vi "checkCmdIdRule.vi"(8 "error in (no error)":errorcluster, 10 "packetConnID":T1, 11 "tcpServer in":refnum<class "TcpServer.lvclass">) -> (0 "error out":errorcluster, 1 "ackIterations":i32, 2 "packetConnID":T1, 3 "tcpServer out":refnum<class "TcpServer.lvclass">)   [LabVIEW 2018, in "TcpServer.lvclass"]
doc: "Get the cmdId sent by TCP Client and compare with lastCmdId saved."
uses:
  TcpServer.lvclass
  typedef/packetConnIDTypeDef.ctl
  TcpServer.lvclass/TcpServer.ctl
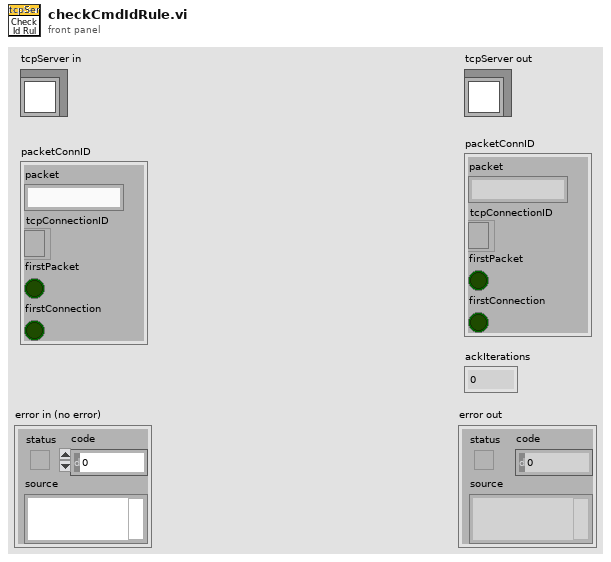
[diagram p1: front panel]
types:
  T1 = typedef "TcpServer.lvclass/packetConnIDTypeDef.ctl" = cluster{"packet":string, "tcpConnectionID":refnum<k5>, "firstPacket":bool, "firstConnection":bool}
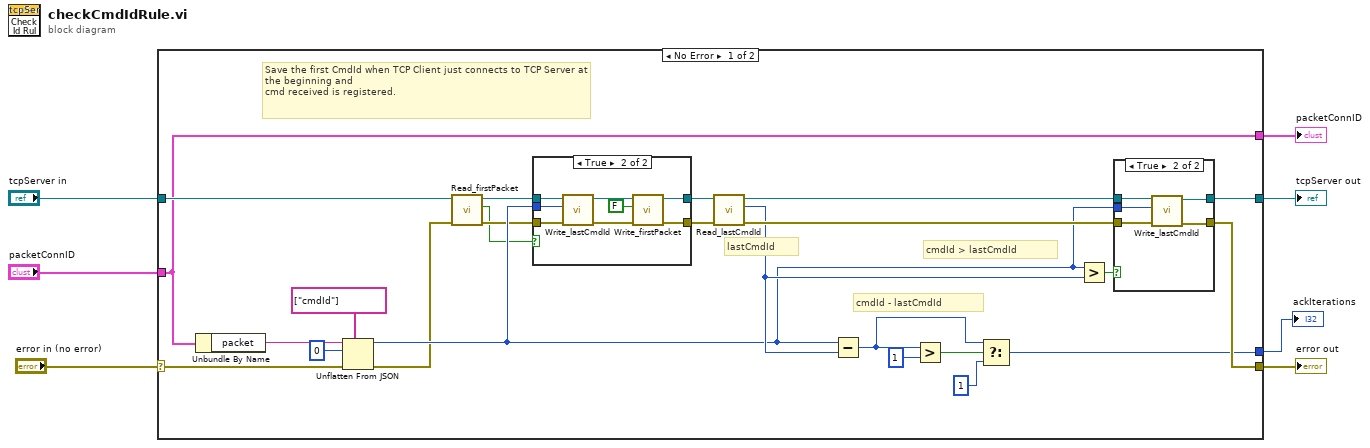
[diagram p0: block diagram]
diagram:
  n1 = case shown="No Error" "error in (no error)" {
    selector: "error in (no error)" -> [w28 w51]
    tunnel: [w25 w51] -> w6
    tunnel: "tcpServer in" -> [w22 w50]
    tunnel: [w27 w50] -> w4
    tunnel: "packetConnID" -> [w18 w49]
    tunnel: [w18 w49] -> w2
    tunnel: [w12 _] -> w1
    frame No Error {
      # "cmdId > lastCmdId"
      # "cmdId - lastCmdId"
      # "Save the first CmdId when TCP Client just connects to TCP Server at the beginning and\ncmd received is registered."
      # "lastCmdId"
      n2 = Unbundle By Name(w18) -> ("packet"=w29:string)
      n3 = Unflatten From JSON(path=string[] ["cmdId"], JSON string=w29, type and defaults=0, error in (no error)=w28) -> (value=w14:i32, error out=w10:errorcluster)  [unwired: 3 in]
      n4 = call "Read_firstPacket.vi"("error in (no error)"=w10, "TcpServer in"=w22) -> ("error out"=w9:errorcluster, "firstPacket"=w8:bool, "TcpServer out"=w11:refnum<class "TcpServer.lvclass">)  [unwired: 7 in]
      n5 = case shown="True" w8 {
        tunnel: w11 -> [w33 w41]
        tunnel: w14 -> [_ w38]
        tunnel: [w33 w35] -> w24
        tunnel: [w32 w37] -> w23
        tunnel: w9 -> [w32 w39]
        frame False {
        }
        frame True {
          n6 = call "Write_lastCmdId.vi"("error in (no error)"=w39, "lastCmdId"=w38, "TcpServer in"=w41) -> ("error out"=w40:errorcluster, "TcpServer out"=w36:refnum<class "TcpServer.lvclass">)  [unwired: 7 in]
          n7 = call "Write_firstPacket.vi"("error in (no error)"=w40, "firstPacket"=FALSE, "TcpServer in"=w36) -> ("error out"=w37:errorcluster, "TcpServer out"=w35:refnum<class "TcpServer.lvclass">)  [unwired: 7 in]
        }
      }
      n8 = call "Read_lastCmdId.vi"("error in (no error)"=w23, "TcpServer in"=w24) -> ("error out"=w26:errorcluster, "lastCmdId"=w15:i32, "TcpServer out"=w19:refnum<class "TcpServer.lvclass">)  [unwired: 7 in]
      n9 = Subtract(x=w14, y=w15) -> (x-y=w16:i32)
      n10 = Greater?(x=w16, y=1) -> (0:w20:bool)
      n11 = Select(t=w16, s=w20, f=1) -> (s? t:f=w12:i32)
      n12 = Greater?(x=w14, y=w15) -> (0:w13:bool)
      n13 = case shown="True" w13 {
        tunnel: w19 -> [w43 w48]
        tunnel: [w43 w47] -> w27
        tunnel: w26 -> [w42 w46]
        tunnel: [w42 w45] -> w25
        tunnel: w14 -> [_ w44]
        frame False {
        }
        frame True {
          n14 = call "Write_lastCmdId.vi"("error in (no error)"=w46, "lastCmdId"=w44, "TcpServer in"=w48) -> ("error out"=w45:errorcluster, "TcpServer out"=w47:refnum<class "TcpServer.lvclass">)  [unwired: 7 in]
        }
      }
    }
    frame Error {
    }
  }
  "error out" <- w6
  "tcpServer out" <- w4
  "packetConnID" <- w2
  "ackIterations" <- w1
